vi "Compute Acceleration.vi"(8 "error in":errorcluster, 10 "AC":waveform(dbl), 11 "DeepU Results in":refnum<class "DeepU Results.lvclass">) -> (0 "error out":errorcluster, 3 "DeepU Results out":refnum<class "DeepU Results.lvclass">)   [LabVIEW 2019, in "Results.lvlib" / "DeepU Results.lvclass"]
uses:
  DeepU Results.lvclass
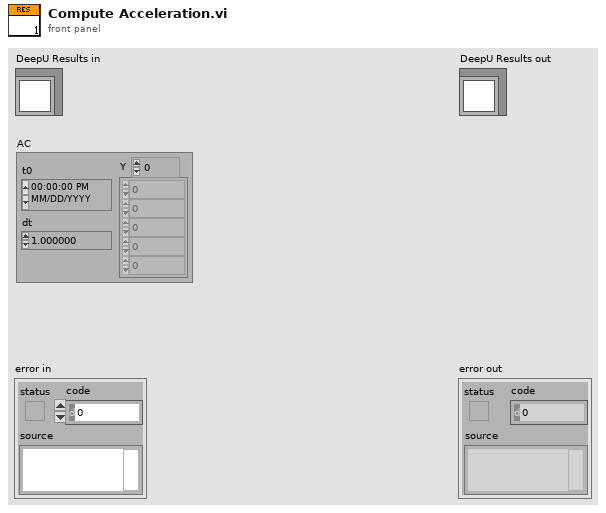
[diagram p1: front panel]
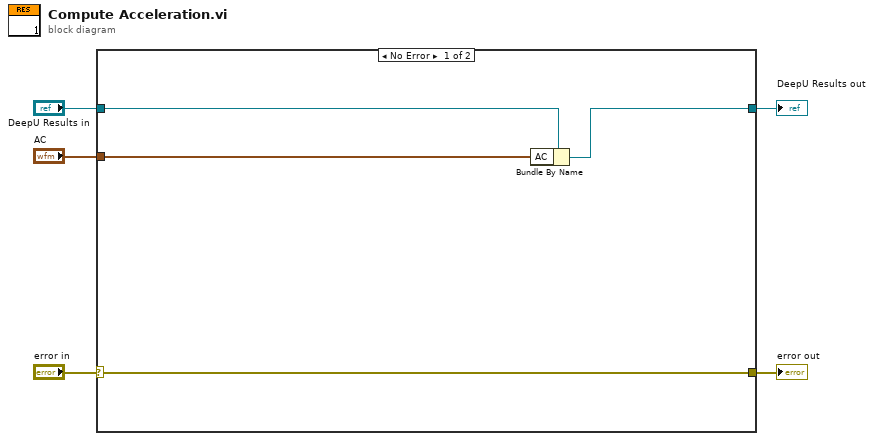
[diagram p0: block diagram]
diagram:
  n1 = case shown="No Error" "error in" {
    selector: "error in" -> [w8 w11]
    tunnel: [w8 w11] -> w4
    tunnel: [w7 w10] -> w2
    tunnel: "DeepU Results in" -> [w9 w10]
    tunnel: "AC" -> [w6 _]
    frame No Error {
      n2 = Bundle By Name(cluster=w9, "AC"=w6) -> (w7:refnum<class "DeepU Results.lvclass">)
    }
    frame Error {
    }
  }
  "error out" <- w4
  "DeepU Results out" <- w2
